vi "turn.vi"(9 "delay":u32, 10 "Carzeta":dbl) -> ()   [LabVIEW 2017]
uses:
  Constant.vi
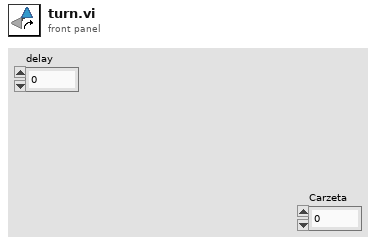
[diagram p1: front panel]
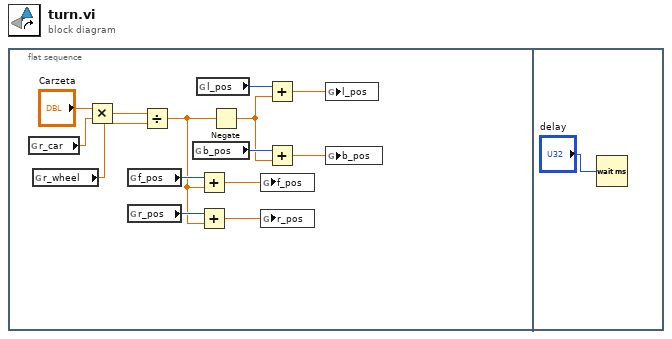
[diagram p0: block diagram]
diagram:
  n1 = flat-sequence {
    frame #0 {
      n2 = global read "Constant.vi" "r_car"() -> (w12:dbl)
      n3 = global read "Constant.vi" "r_wheel"() -> (w11:dbl)
      n4 = Multiply(x="Carzeta", y=w12) -> (x*y=w13:dbl)
      n5 = global read "Constant.vi" "f_pos"() -> (w9:i32)
      n6 = global read "Constant.vi" "r_pos"() -> (w7:i32)
      n7 = Divide(x=w13, y=w11) -> (x/y=w1:dbl)
      n8 = global read "Constant.vi" "b_pos"() -> (w8:i32)
      n9 = global read "Constant.vi" "l_pos"() -> (w10:i32)
      n10 = Add(x=w9, y=w1) -> (x+y=w5:dbl)
      n11 = Add(x=w7, y=w1) -> (x+y=w3:dbl)
      n12 = Negate(x=w1) -> (-x=w2:dbl)
      n13 = global write "Constant.vi" "f_pos"(w5) -> ()
      n14 = global write "Constant.vi" "r_pos"(w3) -> ()
      n15 = Add(x=w10, y=w2) -> (x+y=w6:dbl)
      n16 = Add(x=w8, y=w2) -> (x+y=w4:dbl)
      n17 = global write "Constant.vi" "l_pos"(w6) -> ()
      n18 = global write "Constant.vi" "b_pos"(w4) -> ()
    }
    frame #1 {
      n19 = Wait (ms)(milliseconds to wait="delay") -> ()  [unwired: 1 out]
    }
  }
